vi "Test HIveMQ WebSockets Connection.vi"() -> ()   [LabVIEW 2013]
uses:
  <vilib>/LabVIEW Open Source Project/MQTT Connection/MQTT_Connection/Connection/Connection.lvclass
  <vilib>/LabVIEW Open Source Project/MQTT Websockets Connection/MQTT_Websockets/Connection/WebsocketsConnection.lvclass
panel:
  out "client session error":errorcluster
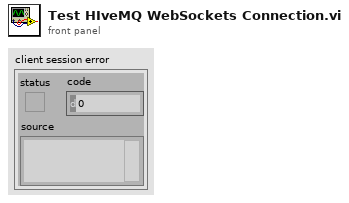
[diagram p1: front panel]
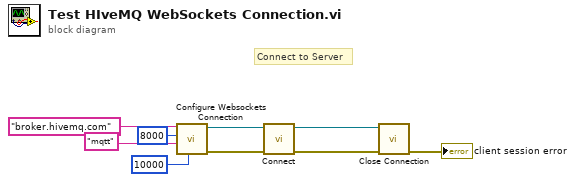
[diagram p0: block diagram]
diagram:
  # "Connect to Server"
  n1 = call <vilib>:"Configure Websockets Connection.vi"("timeout (5000 ms)"=10000 ("timeout (100ms)"), "path"="mqtt", "remote port (80)"=u16 8000, "address (localhost)"="broker.hivemq.com") -> ("error out"=w1:errorcluster, "WSConnection"=w2:refnum<class "WebsocketsConnection.lvclass">)  [unwired: 6 in]
  n2 = call <vilib>:"Connect.vi"("error in (no error)"=w1, "Connection in"=w2) -> ("error out"=w7:errorcluster, "Connection out"=w8:refnum<class "WebsocketsConnection.lvclass">)  [unwired: 8 in]
  n3 = call <vilib>:"Close Connection.vi"("error in (no error)"=w7, "Connection in"=w8) -> ("error out"=→"client session error":errorcluster)  [unwired: 8 in, 1 out]
